vi "Configure DC Voltage Ratio.vi"(0 "VISA resource name":refnum<visa-resource-name>, 1 "NPLC":u16(ring)=1 items=["0.00005", "1", "12", "15"], 2 "Auto Sense Range? (T: Auto)":bool=TRUE, 5 "Auto Range? (T: Auto)":bool, 7 "Manual Range":dbl=1.0, 9 "Aperture Seconds":dbl, 11 "error in (no error)":errorcluster, 13 "Sense Range":u16(ring)=2 items=["0.01", "1", "10"]) -> (4 "VISA resource name out":refnum<visa-resource-name>, 15 "error out":errorcluster)   [LabVIEW 2016, in "Keithley DMM7510.lvlib"]
doc: "This VI configures the DC Voltage ratio measurement and the related parameters."
uses:
  Keithley DMM7510.lvlib
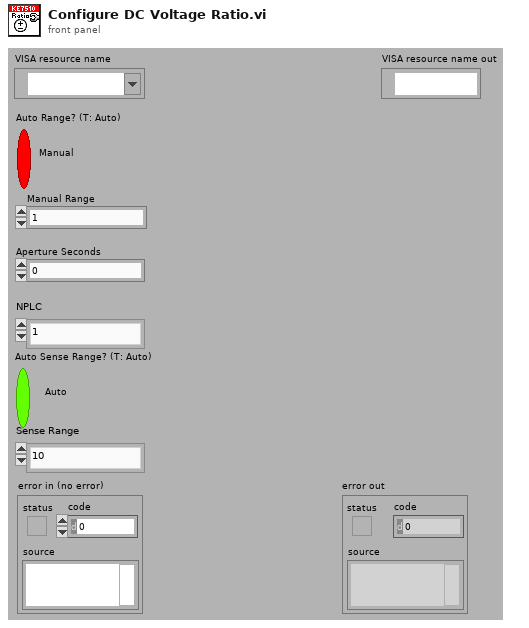
[diagram p1: front panel]
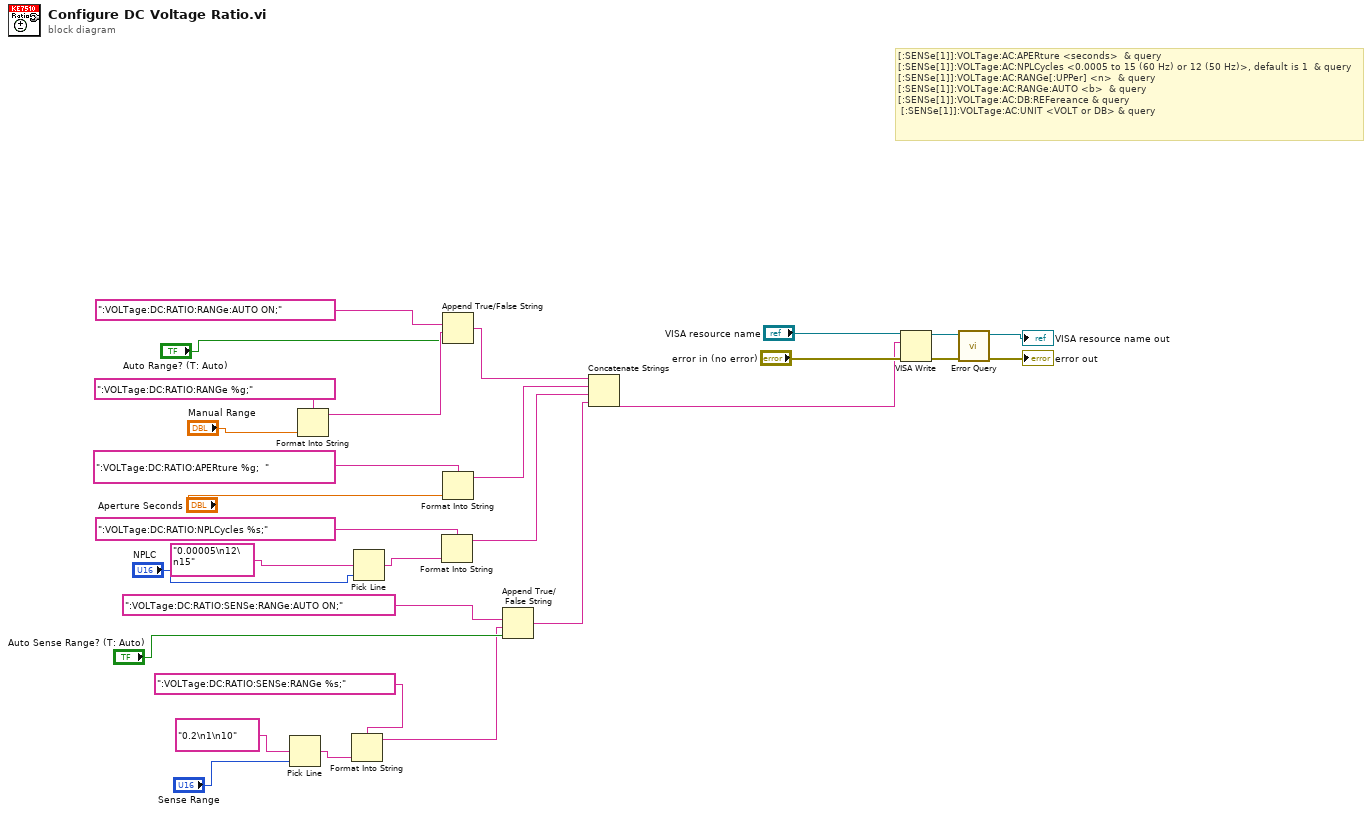
[diagram p0: block diagram]
diagram:
  # "[:SENSe[1]]:VOLTage:AC:APERture <seconds>  & query\n[:SENSe[1]]:VOLTage:AC:NPLCycles <0.0005 to 15 (60 Hz) or 12 (50 Hz)>, default is 1  & query\n[:SENSe[1]]:VOLTage:AC:RANGe[:UPPer] <n>  & query\n[:SENSe[1]]:VOLTage:AC:RANGe:AUTO <b>  & query\n[:SENSe[1]]:VOLTage:AC:DB:REFereance & query\n [:SENSe[1]]:VOLTage:AC:UNIT <VOLT or DB> & query"
  n1 = Pick Line(multi-line string="0.2\n1\n10", line index="Sense Range") -> (output string=w4:string)  [unwired: 1 in]
  n2 = Format Into String(format string=":VOLTage:DC:RATIO:RANGe %g;", "Manual Range") -> (resulting string=w25:string)  [unwired: 2 in, 1 out]
  n3 = Format Into String(format string=":VOLTage:DC:RATIO:SENSe:RANGe %s;", w4) -> (resulting string=w2:string)  [unwired: 2 in, 1 out]
  n4 = Pick Line(multi-line string="0.00005\n12\n15", line index="NPLC") -> (output string=w13:string)  [unwired: 1 in]
  n5 = Format Into String(format string=":VOLTage:DC:RATIO:NPLCycles %s;", w13) -> (resulting string=w20:string)  [unwired: 2 in, 1 out]
  n6 = Append True/False String(1:"Auto Range? (T: Auto)", 2:w25, 3:":VOLTage:DC:RATIO:RANGe:AUTO ON;") -> (0:w22:string)  [unwired: 1 in]
  n7 = Format Into String(format string=":VOLTage:DC:RATIO:APERture %g;  ", "Aperture Seconds") -> (resulting string=w21:string)  [unwired: 2 in, 1 out]
  n8 = Append True/False String(1:"Auto Sense Range? (T: Auto)", 2:w2, 3:":VOLTage:DC:RATIO:SENSe:RANGe:AUTO ON;") -> (0:w1:string)  [unwired: 1 in]
  n9 = Concatenate Strings(w22, w21, w20, w1) -> (w19:string)
  n10 = VISA Write(VISA resource name="VISA resource name", write buffer=w19, error in (no error)="error in (no error)") -> (VISA resource name out=w18:refnum<visa-resource-name>, error out=w17:errorcluster)  [unwired: 1 out]
  n11 = call "Error Query.vi"("error in (no error)"=w17, "VISA resource name"=w18) -> ("error out"=→"error out":errorcluster, "VISA resource name out"=→"VISA resource name out":refnum<visa-resource-name>)  [unwired: 6 in, 2 out]
